vi "Heat2D_X Neumann RHS.vi"(8 "BC Value(n)":dbl[](array[numeric]), 9 "Left?":bool, 10 "Extended U(n)":dbl[][](array[numeric]), 11 "Coefficients":T1) -> (3 "RHS vector":dbl[](array[numeric]))   [LabVIEW 2020, in "NI_PDE.lvlib"]
uses:
  <vilib>/gmath/NI_PDE.lvlib
  <vilib>/Analysis/2dsp.llb/2D Convolution (DBL).vi
  <vilib>/Analysis/NI_AALPro.lvlib
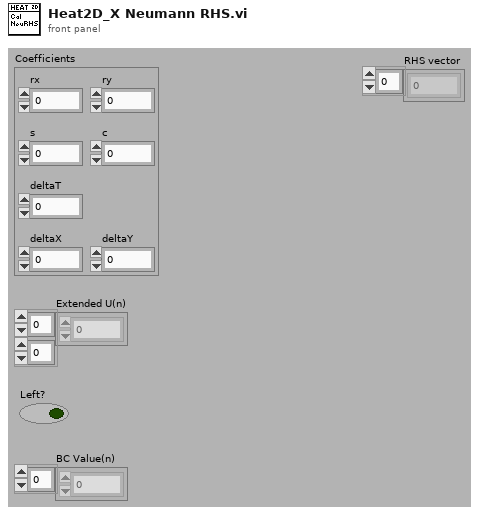
[diagram p1: front panel]
types:
  T1 = cluster{"rx":dbl, "ry":dbl, "s":dbl, "c":dbl, "deltaT":dbl, "deltaX":dbl, "deltaY":dbl}
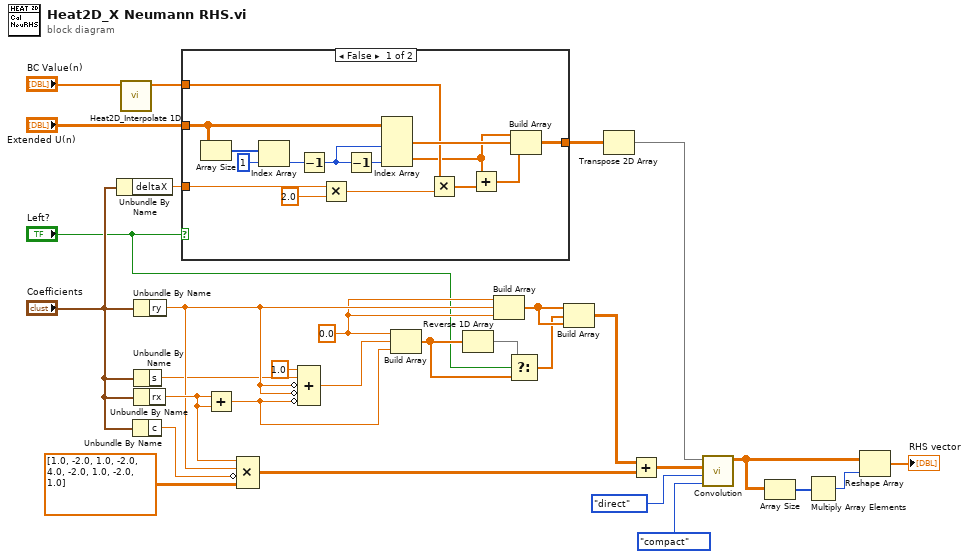
[diagram p0: block diagram]
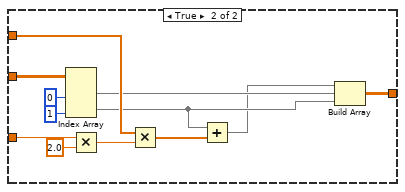
[diagram p2: hidden frame]
diagram:
  w16 = 0.0 ("element")
  n1 = Unbundle By Name("Coefficients") -> ("deltaX"=w6:dbl)
  n2 = call <vilib>:"Heat2D_Interpolate 1D.vi"("X"="BC Value(n)") -> ("Interp(X)"=w2:dbl[])  [unwired: 1 in, 9 out]
  n3 = Unbundle By Name("Coefficients") -> ("c"=w25:dbl)
  n4 = Unbundle By Name("Coefficients") -> ("ry"=w23:dbl)
  n5 = Unbundle By Name("Coefficients") -> ("s"=w19:dbl)
  n6 = Unbundle By Name("Coefficients") -> ("rx"=w24:dbl)
  n7 = case shown="False" "Left?" {
    tunnel: "Extended U(n)" -> [w41 w47]
    tunnel: [w45 w55] -> w8
    tunnel: w2 -> [w35 w51]
    tunnel: w6 -> [w36 w54]
    frame False {
      n8 = Array Size(array=w41) -> (size(s)=w42:i32[])
      n9 = Index Array(array=w42, index=1) -> (element=w40:i32)
      n10 = Decrement(x=w40) -> (x-1=w31:i32)
      n11 = Multiply(x=w36, y=2.0) -> (x*y=w37:dbl)
      n12 = Decrement(x=w31) -> (x-1=w39:i32)
      n13 = Index Array(array=w41, index (col) #1=w31, index (col) #2=w39) -> (element #1=w44:dbl[], element #2=w33:dbl[])  [unwired: 2 in]
      n14 = Multiply(x=w35, y=w37) -> (x*y=w34:dbl[])
      n15 = Add(x=w33, y=w34) -> (x+y=w32:dbl[])
      n16 = Build Array(w33, w44, w32) -> (w45:dbl[][])
    }
    frame True {
      n17 = Index Array(array=w47, index (col) #1=0 ("disabled index (col)"), index (col) #2=1 ("index (col)")) -> (element #1=w48:dbl[], element #2=w49:dbl[])  [unwired: 2 in]
      n18 = Multiply(x=w54, y=2.0) -> (x*y=w52:dbl)
      n19 = Multiply(x=w51, y=w52) -> (x*y=w50:dbl[])
      n20 = Add(x=w49, y=w50) -> (x+y=w46:dbl[])
      n21 = Build Array(w46, w48, w49) -> (w55:dbl[][])
    }
  }
  n22 = Add(x=w24, y=w24) -> (x+y=w17:dbl)
  n23 = Compound Arithmetic op=MULTIPLY(w24, w23, invert w25, dbl[][] [[1.0, -2.0, 1.0], [-2.0, 4.0, -2.0], [1.0, -2.0, 1.0]]) -> (w13:dbl[][])
  n24 = Compound Arithmetic op=ADD(1.0 ("value"), w19, invert w23, invert w23, invert w17) -> (w22:dbl)
  n25 = Build Array(w16, w22, w17) -> (w14:dbl[])
  n26 = Reverse 1D Array(array=w14) -> (reversed array=w15:dbl[])
  n27 = Build Array(w16, w23, w16) -> (w21:dbl[])
  n28 = Select(t=w15, s="Left?", f=w14) -> (s? t:f=w18:dbl[])
  n29 = Build Array(w21, w18, w21) -> (w26:dbl[][])
  n30 = Transpose 2D Array(2D array=w8) -> (transposed array=w1:dbl[][])
  n31 = Add(x=w26, y=w13) -> (x+y=w27:dbl[][])
  n32 = call-poly <vilib>:"Convolution.vi"("output size"=enum32{"full", "size X", "compact"}."compact", "algorithm"=enum32{"direct", "frequency domain"}."direct", "Y"=w27, "X"=w1) -> ("X * Y"=w28:dbl[][])  [unwired: 7 out]
  n33 = Array Size(array=w28) -> (size(s)=w12:i32[])
  n34 = Multiply Array Elements(1:w12) -> (0:w29:i32)
  n35 = Reshape Array(w28, w29) -> (→"RHS vector":dbl[])
